vi "changeRowColor.vi"() -> ()   [LabVIEW 2012]
uses:
  <vilib>/Utility/miscctls.llb/LVRowAndColumnTypeDef.ctl
  <vilib>/addons/database/Connection.llb/DB Tools Open Connec (Path).vi
  <vilib>/addons/database/_DB Variant To Data/Database Variant To Data.xnode
  <vilib>/addons/database/NI_Database_API.lvlib
panel:
  in  "Active Cell:Active Cell":T1
  in  "Running":string[][](table)
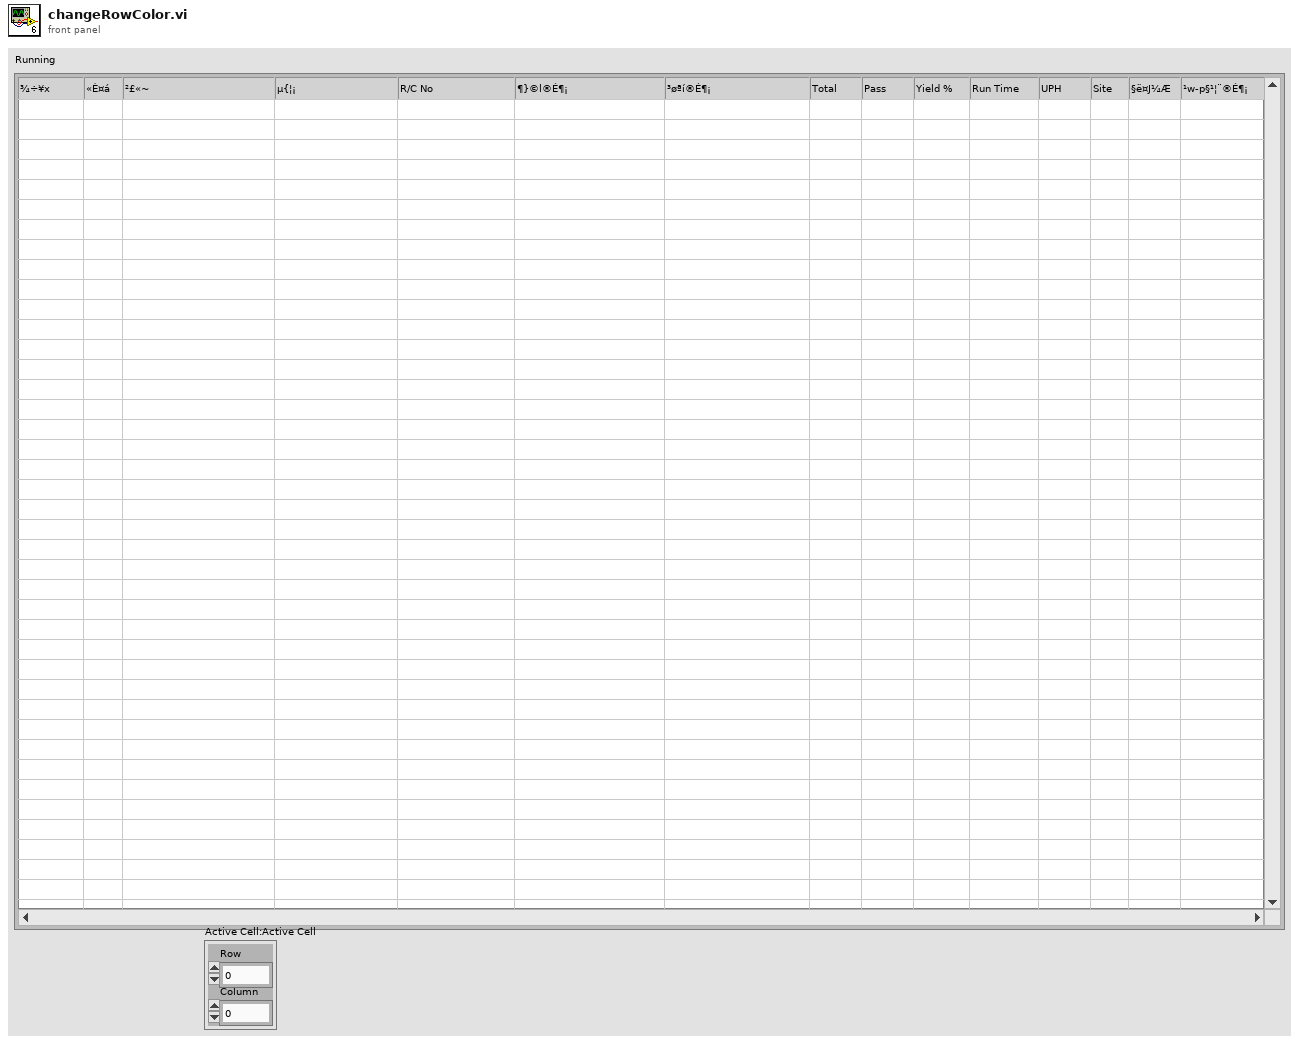
[diagram p1: front panel]
types:
  T1 = typedef "LVRowAndColumnTypeDef.ctl" = cluster{"Row":i32, "Column":i32}
  T2 = typedef "NI_Database_API.lvlib/Conn ObjectReference.ctl" = refnum<k1>
  T3 = typedef "LVDateTimeRec.ctl" = cluster{"fractional second":dbl, "second":i32, "minute":i32, "hour":i32, "day of month":i32, "month":i32, "year":i32, "day of week":i32, "day of year":i32, "DST":i32}
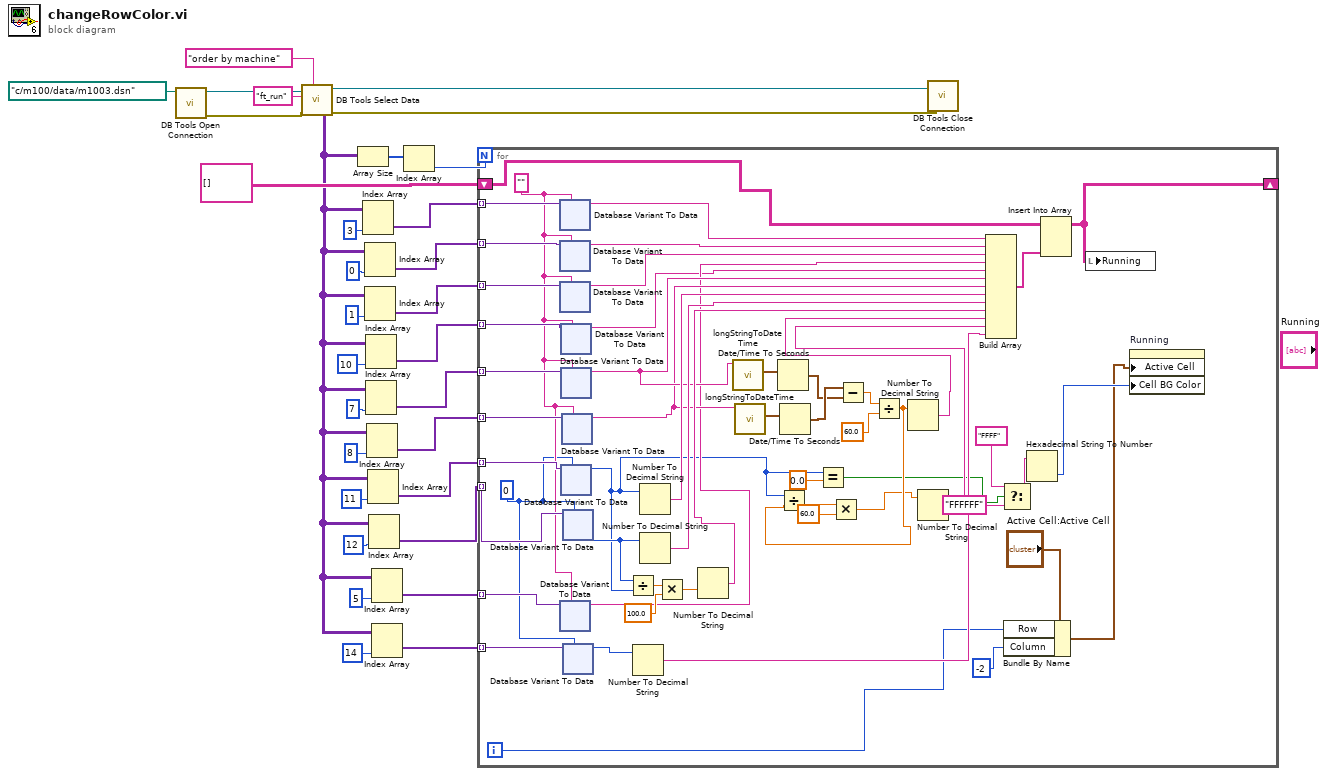
[diagram p0: block diagram]
diagram:
  n1 = call-poly <vilib>:"DB Tools Open Connection.vi"("connection information"=path "c:/m100/data/m1003.dsn") -> ("error out"=w30:errorcluster, "connection reference"=w31:T2)  [unwired: 7 in]
  n2 = call <vilib>:"DB Tools Select Data.vi"("condition"="order by machine", "error in (no error)"=w30, "table"="ft_run", "connection reference"=w31) -> ("error out"=w28:errorcluster, "data"=w4:variant[][], "connection reference out"=w29:T2)  [unwired: 2 in]
  n3 = Array Size(array=w4) -> (size(s)=w25:i32[])
  n4 = Index Array(array=w4, index (col)=3) -> (element=w14:variant[])  [unwired: 1 in]
  n5 = Index Array(array=w4, index (col)=0) -> (element=w21:variant[])  [unwired: 1 in]
  n6 = Index Array(array=w4, index (col)=1) -> (element=w13:variant[])  [unwired: 1 in]
  n7 = Index Array(array=w4, index (col)=10) -> (element=w12:variant[])  [unwired: 1 in]
  n8 = Index Array(array=w4, index (col)=7) -> (element=w11:variant[])  [unwired: 1 in]
  n9 = Index Array(array=w4, index (col)=8) -> (element=w7:variant[])  [unwired: 1 in]
  n10 = Index Array(array=w4, index (col)=11) -> (element=w10:variant[])  [unwired: 1 in]
  n11 = Index Array(array=w4, index (col)=12) -> (element=w9:variant[])  [unwired: 1 in]
  n12 = Index Array(array=w4, index (col)=5) -> (element=w5:variant[])  [unwired: 1 in]
  n13 = Index Array(array=w4, index (col)=14 ("disabled index (col)")) -> (element=w2:variant[])  [unwired: 1 in]
  n14 = Index Array(array=w25) -> (element=w24:i32)  [unwired: 1 in]
  n15 = for {
    N: w24 -> [_]
    tunnel: w21 -> [w80] mode=indexing
    tunnel: w9 -> [w85] mode=indexing
    shift-right: [w82] -> _
    shift-left: string[][] [] -> [w84]
    tunnel: w14 -> [w81] mode=indexing
    tunnel: w13 -> [w79] mode=indexing
    tunnel: w12 -> [w78] mode=indexing
    tunnel: w11 -> [w77] mode=indexing
    tunnel: w10 -> [w76] mode=indexing
    tunnel: w7 -> [w71] mode=indexing
    tunnel: w5 -> [w54] mode=indexing
    tunnel: w2 -> [w48] mode=indexing
    i -> [w39]
    w47 = 0
    w53 = ""
    n16 = xnode "Database Variant To Data"("database variant"=w81, "type"=w53) -> ("data"=w52:string)  [unwired: 1 in, 1 out]
    n17 = xnode "Database Variant To Data"("database variant"=w80, "type"=w53) -> ("data"=w51:string)  [unwired: 1 in, 1 out]
    n18 = xnode "Database Variant To Data"("database variant"=w79, "type"=w53) -> ("data"=w50:string)  [unwired: 1 in, 1 out]
    n19 = xnode "Database Variant To Data"("database variant"=w54, "type"=w53) -> ("data"=w49:string)  [unwired: 1 in, 1 out]
    n20 = xnode "Database Variant To Data"("database variant"=w78, "type"=w53) -> ("data"=w43:string)  [unwired: 1 in, 1 out]
    n21 = xnode "Database Variant To Data"("database variant"=w77, "type"=w53) -> ("data"=w67:string)  [unwired: 1 in, 1 out]
    n22 = xnode "Database Variant To Data"("database variant"=w76, "type"=w47) -> ("data"=w36:i32)  [unwired: 1 in, 1 out]
    n23 = xnode "Database Variant To Data"("database variant"=w71, "type"=w53) -> ("data"=w66:string)  [unwired: 1 in, 1 out]
    n24 = xnode "Database Variant To Data"("database variant"=w85, "type"=w47) -> ("data"=w75:i32)  [unwired: 1 in, 1 out]
    n25 = xnode "Database Variant To Data"("database variant"=w48, "type"=w47) -> ("data"=w46:i32)  [unwired: 1 in, 1 out]
    n26 = Divide(x=w75, y=w36) -> (x/y=w72:dbl)
    n27 = Number To Decimal String(number=w46) -> (decimal integer string=w45:string)  [unwired: 1 in]
    n28 = Number To Decimal String(number=w36) -> (decimal integer string=w70:string)  [unwired: 1 in]
    n29 = Number To Decimal String(number=w75) -> (decimal integer string=w69:string)  [unwired: 1 in]
    n30 = Multiply(x=w72, y=100.0) -> (x*y=w73:dbl)
    n31 = Number To Decimal String(number=w73) -> (decimal integer string=w68:string)  [unwired: 1 in]
    n32 = call "longStringToDateTime.vi"("input string"=w67) -> ("output cluster"=w64:T3)  [unwired: 10 in]
    n33 = call "longStringToDateTime.vi"("input string"=w66) -> ("output cluster"=w65:T3)  [unwired: 10 in]
    n34 = Date/Time To Seconds(2:w64) -> (0:w62:timestamp)  [unwired: 1 in]
    n35 = Date/Time To Seconds(2:w65) -> (0:w63:timestamp)  [unwired: 1 in]
    n36 = Equal?(x=w36, y=0.0) -> (x = y?=w35:bool)
    n37 = Subtract(x=w63, y=w62) -> (x-y=w61:dbl)
    n38 = Divide(x=w61, y=60.0) -> (x/y=w58:dbl)
    n39 = Divide(x=w36, y=w58) -> (x/y=w57:dbl)
    n40 = Multiply(x=w57, y=60.0) -> (x*y=w44:dbl)
    n41 = Number To Decimal String(number=w58) -> (decimal integer string=w59:string)  [unwired: 1 in]
    n42 = Number To Decimal String(number=w44) -> (decimal integer string=w55:string)  [unwired: 1 in]
    n43 = Build Array(w52, w51, w50, w49, w43, w67, w66, w70, w69, w68, w59, w55, w45) -> (w83:string[])
    n44 = Select(t="FFFF" ("string"), s=w35, f="FFFFFF") -> (s? t:f=w33:string)
    n45 = Bundle By Name(cluster="Active Cell:Active Cell", "Row"=w39, "Column"=-2 ("element")) -> (w38:T1)
    n46 = Hexadecimal String To Number(string=w33) -> (number=w42:u32)  [unwired: 2 in, 1 out]
    n47 = Insert Into Array(array=w84, new element=w83) -> (w82:string[][])  [unwired: 2 in]
    n48 = local write "Running"(w82) -> ()
    n49 = property on="Running" class="Tbl (strict)"("Active Cell"=w38, "Cell BG Color"=w42) -> ()  [unwired: 2 in, 2 out]
  }
  n50 = call <vilib>:"DB Tools Close Connection.vi"("error in (no error)"=w28, "connection reference"=w29) -> ()  [unwired: 5 in, 1 out]
